vi "Read Value.vi"(8 "error in (no error)":errorcluster, 11 "fixed32 in":refnum<class "string.lvclass">) -> (0 "error out":errorcluster, 2 "Value":string, 3 "fixed32 out":refnum<class "string.lvclass">)   [LabVIEW 2020, in "Protobuf RAW.lvlib" / "string.lvclass"]
uses:
  string.lvclass
  string.lvclass/string.ctl
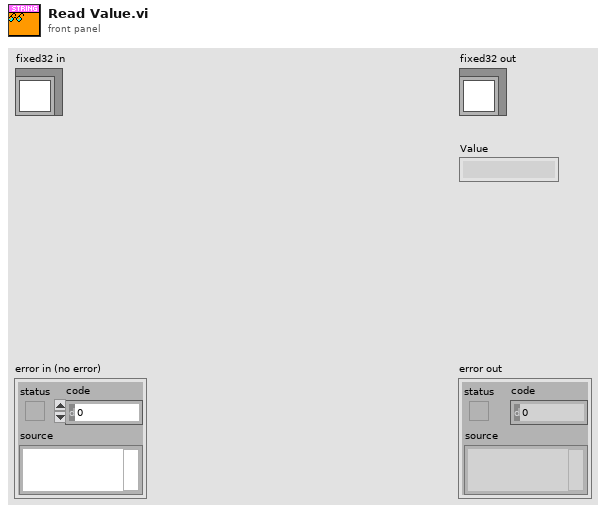
[diagram p1: front panel]
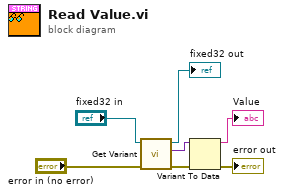
[diagram p0: block diagram]
diagram:
  n1 = call-dynamic "Get Variant.vi"("error in (no error)"="error in (no error)", "Proto Type Common in"="fixed32 in") -> ("error out"=w6:errorcluster, "Value"=w2:variant, "Proto Type Common out"=→"fixed32 out":refnum<class "string.lvclass">)  [unwired: 7 in]
  n2 = Variant To Data(error in=w6, Variant=w2) -> (data=→"Value":string, error out=→"error out":errorcluster)  [unwired: 1 in]
